vi "WaveformReader.vi"() -> ()   [LabVIEW 2020]
doc: "Copyright © 2008 - 2024 VI Technologies B.V. \nALL RIGHTS RESERVED"
uses:
  SuperNS/StreamStatus.ctl
  SuperNS/SuperNS.lvclass
  WaveFormData/WfmData.lvclass
panel:
  out "StreamStatus":T1
  out "error out":errorcluster
  out "My IP address":string
  out "Waveform Graph":waveform(dbl)(graph)
  in  "My Name":string="DataReader"
  in  "Writer URL":string
  # "Waveform reader"
  # "Copyright (c) 2024, VI Technologies B.V.\nAll rights reserved.\n\nRedistribution and use in source and binary forms, with or without modification, are permitted provided that \nthe following conditions are met:\n\n * Redistributions of source code must retain the above copyright notice, this list of conditions and the \nfollowing disclaimer.\n * Redistributions in binary form must reproduce the above copyright notice, this list of conditions and the \nfollowing disclaimer in the documentation and/or other materials provided with the distribution.\n * Neither the name of VI Technologies B.V. nor the names of its contributors may be used to endorse or \npromote products derived from this software without specific prior written permission.\n\nTHIS SOFTWARE IS PROVIDED BY THE COPYRIGHT HOLDERS AND CONTRIBUTORS \"AS IS\" AND ANY EXPRESS OR \nIMPLIED WARRANTIES, INCLUDING, BUT NOT LIMITED TO, THE IMPLIED WARRANTIES OF MERCHANTABILITY \nAND FITNESS FOR A PARTICULAR PURPOSE ARE DISCLAIMED. IN NO EVENT SHALL THE COPYRIGHT OWNER OR \nCONTRIBUTORS BE LIABLE FOR ANY DIRECT, INDIRECT, INCIDENTAL, SPECIAL, EXEMPLARY, OR CONSEQUENTIAL \nDAMAGES (INCLUDING, BUT NOT LIMITED TO, PROCUREMENT OF SUBSTITUTE GOODS OR SERVICES; LOSS OF \nUSE, DATA, OR PROFITS; OR BUSINESS INTERRUPTION) HOWEVER CAUSED AND ON ANY THEORY OF LIABILITY, \nWHETHER IN CONTRACT, STRICT LIABILITY, OR TORT (INCLUDING NEGLIGENCE OR OTHERWISE) ARISING IN ANY \nWAY OUT OF THE USE OF THIS SOFTWARE, EVEN IF ADVISED OF THE POSSIBILITY OF SUCH DAMAGE.\n\nFor more information, please visit https://www.vi-tech.nl or contact us at info@vi-tech.nl"
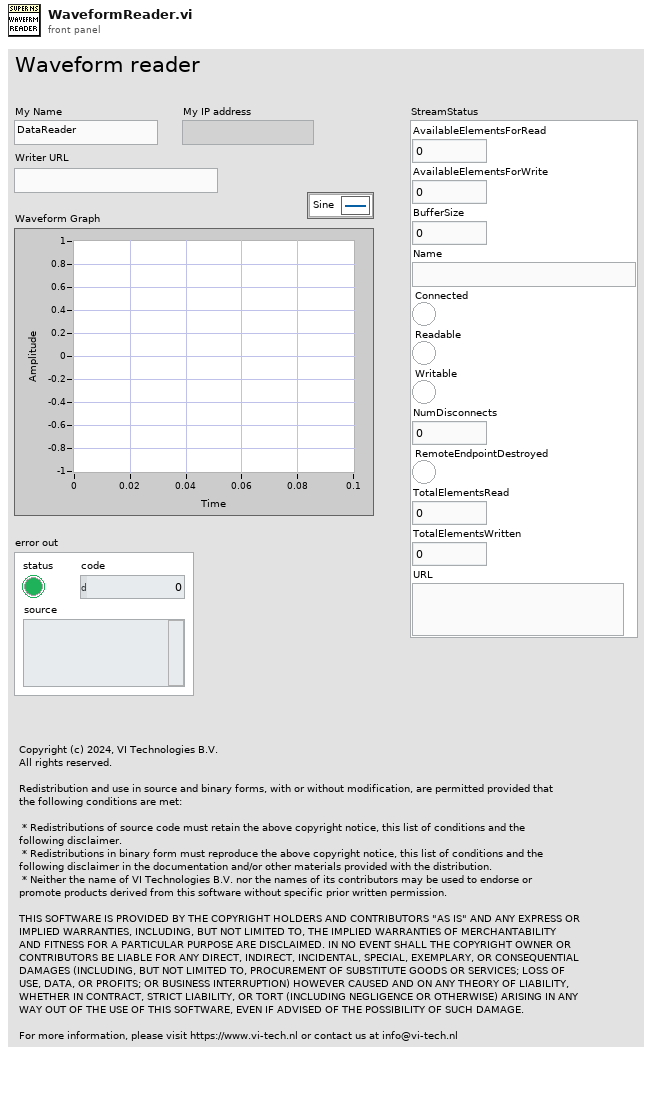
[diagram p1: front panel]
types:
  T1 = typedef "SuperNS.lvclass/StreamStatus.ctl" = cluster{"AvailableElementsForRead":i32, "AvailableElementsForWrite":i32, "BufferSize":i32, "Name":string, "Connected":bool, "Readable":bool, "Writable":bool, "NumDisconnects":u32, "RemoteEndpointDestroyed":bool, "TotalElementsRead":u64, "TotalElementsWritten":u64, "URL":string}
  T2 = typedef "SuperNS.lvclass/StreamDataType.ctl" = refnum<class>
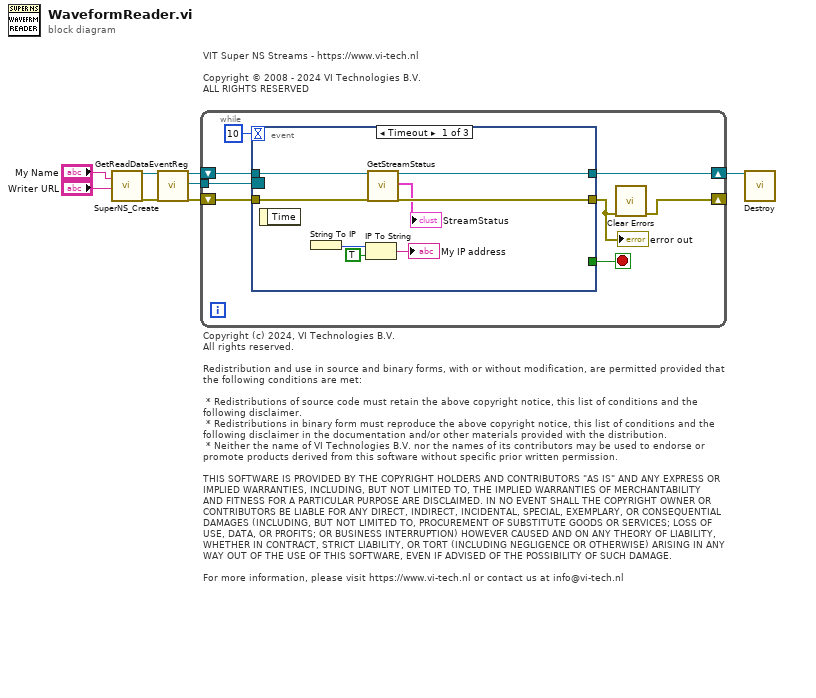
[diagram p0: block diagram]
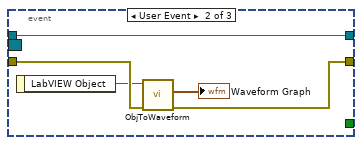
[diagram p2: hidden frame]
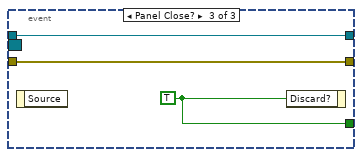
[diagram p3: hidden frame]
diagram:
  # "VIT Super NS Streams - https://www.vi-tech.nl\n\nCopyright © 2008 - 2024 VI Technologies B.V. \nALL RIGHTS RESERVED"
  # "Copyright (c) 2024, VI Technologies B.V.\nAll rights reserved.\n\nRedistribution and use in source and binary forms, with or without modification, are permitted provided that \nthe following conditions are met:\n\n * Redistributions of source code must retain the above copyright notice, this list of conditions and the \nfollowing disclaimer.\n * Redistributions in binary form must reproduce the above copyright notice, this list of conditions and the \nfollowing disclaimer in the documentation and/or other materials provided with the distribution.\n * Neither the name of VI Technologies B.V. nor the names of its contributors may be used to endorse or \npromote products derived from this software without specific prior written permission.\n\nTHIS SOFTWARE IS PROVIDED BY THE COPYRIGHT HOLDERS AND CONTRIBUTORS \"AS IS\" AND ANY EXPRESS OR \nIMPLIED WARRANTIES, INCLUDING, BUT NOT LIMITED TO, THE IMPLIED WARRANTIES OF MERCHANTABILITY \nAND FITNESS FOR A PARTICULAR PURPOSE ARE DISCLAIMED. IN NO EVENT SHALL THE COPYRIGHT OWNER OR \nCONTRIBUTORS BE LIABLE FOR ANY DIRECT, INDIRECT, INCIDENTAL, SPECIAL, EXEMPLARY, OR CONSEQUENTIAL \nDAMAGES (INCLUDING, BUT NOT LIMITED TO, PROCUREMENT OF SUBSTITUTE GOODS OR SERVICES; LOSS OF \nUSE, DATA, OR PROFITS; OR BUSINESS INTERRUPTION) HOWEVER CAUSED AND ON ANY THEORY OF LIABILITY, \nWHETHER IN CONTRACT, STRICT LIABILITY, OR TORT (INCLUDING NEGLIGENCE OR OTHERWISE) ARISING IN ANY \nWAY OUT OF THE USE OF THIS SOFTWARE, EVEN IF ADVISED OF THE POSSIBILITY OF SUCH DAMAGE.\n\nFor more information, please visit https://www.vi-tech.nl or contact us at info@vi-tech.nl"
  n1 = call "SuperNS_Create.vi"("NSName"="My Name", "RemoteEP_URL"="Writer URL") -> ("SuperNS Reference"=w1:refnum<class "SuperNS.lvclass">, "error out"=w7:errorcluster)  [unwired: 16 in]
  n2 = call-dynamic "GetReadDataEventReg.vi"("reference in"=w1, "error in"=w7) -> ("reference out"=w5:refnum<class "SuperNS.lvclass">, "SuperNS ReadData"=w4:refnum<event-registration>, "error out"=w8:errorcluster)  [unwired: 15 in]
  n3 = while {
    shift-right: [w12] -> w6
    shift-left: w5 -> [w13]
    tunnel: w4 -> [w11]
    shift-right: [w15] -> _
    shift-left: w8 -> [w16]
    stop <- w14 stop-if-true
    n4 = event shown="[0] Timeout" {
      selector: w11 -> [_ _ _]
      dyn-events: _ -> [_ _ _]
      timeout: 10 -> [_ _ _]
      tunnel: [_ _ w32] -> w14
      tunnel: w13 -> [w18 w26 w31]
      tunnel: [w19 w26 w31] -> w12
      tunnel: w16 -> [w23 w29 w30]
      tunnel: [w24 w28 w30] -> w9
      event Timeout {
        n5 = event-data() -> ()  [unwired: 1 in, 1 out]
        n6 = String To IP() -> (0:w20:u32)  [unwired: 1 in]
        n7 = IP To String(1:TRUE ("dot notation? (F)"), 2:w20) -> (0:→"My IP address":string)
        n8 = call-dynamic "GetStreamStatus.vi"("reference in"=w18, "error in"=w23) -> ("reference out"=w19:refnum<class "SuperNS.lvclass">, "StreamStatus"=→"StreamStatus":T1, "error out"=w24:errorcluster)  [unwired: 13 in, 2 out]
      }
      event User Event {
        n9 = event-data() -> ("LabVIEW Object"=w27:T2)  [unwired: 1 in]
        n10 = call "ObjToWaveform.vi"("error in"=w29, "LabVIEW Object"=w27) -> ("error out"=w28:errorcluster, "Waveform"=→"Waveform Graph":waveform(dbl))  [unwired: 8 in]
      }
      event Panel Close? {
        w32 = TRUE ("Discard?")
        n11 = event-data() -> ()  [unwired: 1 in, 1 out]
        n12 = event-data("Discard?"=w32) -> ()  [unwired: 1 in, 1 out]
      }
    }
    "error out" <- w9
    n13 = call <vilib>:"Clear Errors.vi"("error in (no error)"=w9) -> ("error out"=w15:errorcluster)  [unwired: 5 in, 1 out]
  }
  n14 = call-dynamic "Destroy.vi"("reference in"=w6) -> ()  [unwired: 17 in, 2 out]
